vi "Get Solar Angles.vi"(9 "lattitude":dbl, 10 "Numeric 3":dbl, 11 "TST (min)":dbl) -> (1 "Solar Zenith Angle (deg)":dbl, 2 "Solar Elevation Angle (deg)":dbl, 3 "Hous Angle (deg)":dbl)   [LabVIEW 2013, in "Solar Calculations.lvlib"]
uses:
  Solar Calculations.lvlib
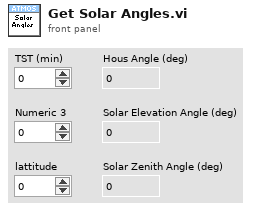
[diagram p1: front panel]
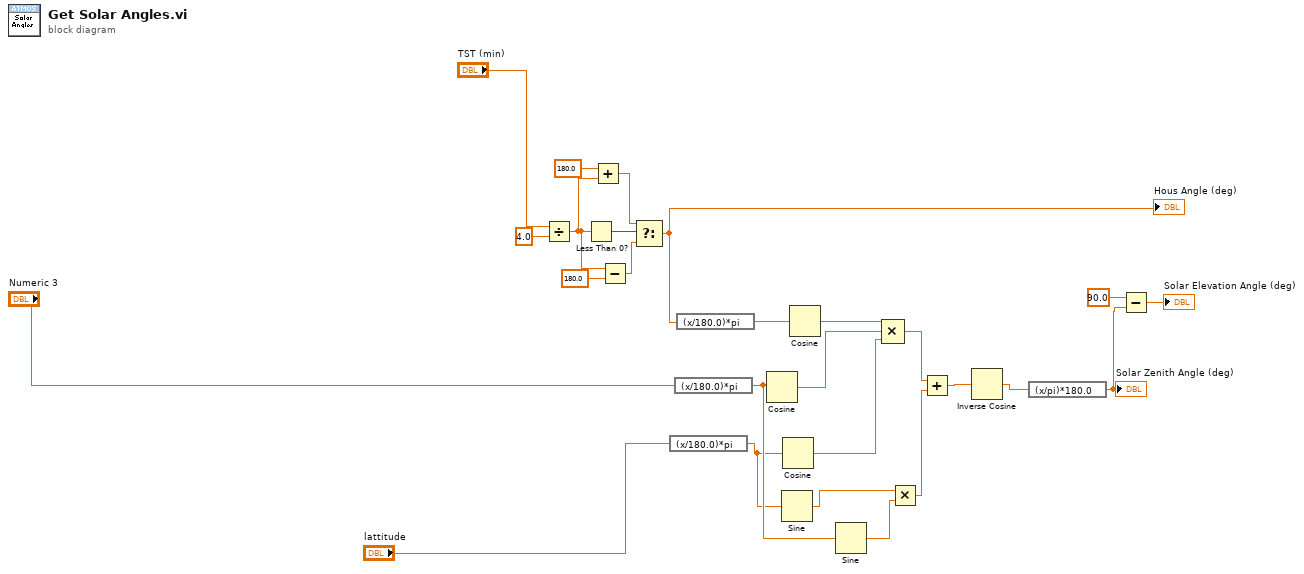
[diagram p0: block diagram]
diagram:
  n1 = Divide(x="TST (min)", y=4.0) -> (x/y=w5:dbl)
  n2 = Less Than 0?(x=w5) -> (x < 0?=w3:bool)
  n3 = Add(x=180.0, y=w5) -> (x+y=w8:dbl)
  n4 = Subtract(x=w5, y=180.0) -> (x-y=w7:dbl)
  n5 = Select(t=w8, s=w3, f=w7) -> (s? t:f=w9:dbl)
  "Hous Angle (deg)" <- w9
  n6 = expression code="(x/180.0)*pi" ("degrees to radians")("lattitude") -> (w16:dbl)
  n7 = expression code="(x/180.0)*pi" ("degrees to radians")("Numeric 3") -> (w17:dbl)
  n8 = expression code="(x/180.0)*pi" ("degrees to radians")(w9) -> (w10:dbl)
  n9 = Cosine(x=w17) -> (cos(x)=w14:dbl)
  n10 = Sine(x=w16) -> (sin(x)=w18:dbl)
  n11 = Cosine(x=w16) -> (cos(x)=w15:dbl)
  n12 = Cosine(x=w10) -> (cos(x)=w13:dbl)
  n13 = Sine(x=w17) -> (sin(x)=w19:dbl)
  n14 = Compound Arithmetic op=MULTIPLY(w13, w14, w15) -> (w20:dbl)
  n15 = Multiply(x=w18, y=w19) -> (x*y=w21:dbl)
  n16 = Add(x=w20, y=w21) -> (x+y=w22:dbl)
  n17 = Inverse Cosine(1:w22) -> (0:w23:dbl)
  n18 = expression code="(x/pi)*180.0" ("radians to degrees")(w23) -> (w25:dbl)
  "Solar Zenith Angle (deg)" <- w25
  n19 = Subtract(x=90.0, y=w25) -> (x-y=→"Solar Elevation Angle (deg)":dbl)
